vi "Alias.vi"() -> ()   [LabVIEW 2024]
uses:
  ASW/Source/DigitalThreadServices/DataStoreClient.LabVIEW/source/API/Metadata/Extension.ctl
  ASW/Source/DigitalThreadServices/DataStoreClient.LabVIEW/source/API/Metadata/NI Metadata Types.lvlib
  ASW/Source/DigitalThreadServices/DataStoreClient.LabVIEW/source/API/Metadata/Operator.ctl
  ASW/Source/DigitalThreadServices/DataStoreClient.LabVIEW/source/API/Metadata Store V1/NI Metadata Store V1 Client.lvlib
  ASW/Source/DigitalThreadServices/DataStoreClient.LabVIEW/source/API/Data Store V1/NI Data Store V1 Client.lvlib
  ASW/Source/DigitalThreadServices/DataStoreClient.LabVIEW/source/API/Metadata/Outcome.ctl
  ASW/Source/DigitalThreadServices/DataStoreClient.LabVIEW/source/API/Data Store V1/Test Result.ctl
  ASW/Source/DigitalThreadServices/DataStoreClient.LabVIEW/source/API/Metadata/Alias Target Type.ctl
  ASW/Source/DigitalThreadServices/DataStoreClient.LabVIEW/source/API/Metadata Store V1/Create Alias (Metadata - Operator).vi
  ASW/Source/DigitalThreadServices/DataStoreClient.LabVIEW/source/API/Metadata Store V1/Create Operator.vi
  ASW/Source/DigitalThreadServices/DataStoreClient.LabVIEW/source/API/Metadata Store V1/Get Operator.vi
  ASW/Source/DigitalThreadServices/DataStoreClient.LabVIEW/source/API/Metadata/Error Information.ctl
  ASW/Source/DigitalThreadServices/DataStoreClient.LabVIEW/source/API/Metadata/Alias.ctl
panel:
  in  "Operator Info":cluster{"Name":string, "Alias":string}[](array[cluster])=[{"Name"="Jane Doe", "Alias"="primary_operator"}, {"Name"="John Smith", "Alias"="secondary_operator"}]
  out "query aliases results":T1[](array[typedef])
  out "get alias results":T1
  out "log":string
  out "error out":errorcluster
  # "Using Aliases\n\nThis example shows how to use the datastore API to...\n- Create aliases for metadata\n- Use created aliases\n- Retrieve aliases\n- Delete aliases"
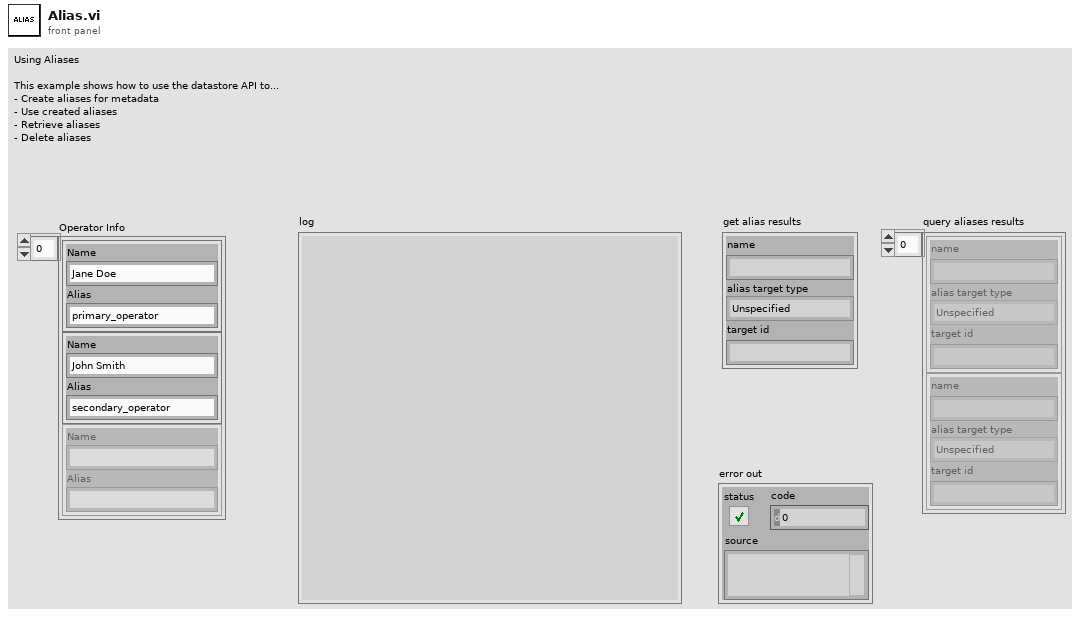
[diagram p1: front panel]
types:
  T1 = typedef "NI Metadata Types.lvlib/Alias.ctl" = cluster{"name":string, "alias target type":T2, "target id":string}
  T2 = typedef "NI Metadata Types.lvlib/Alias Target Type.ctl" = enum32{"Unspecified", "UUT Instance", "UUT", "Hardware Item", "Software Item", "Operator", "Test Description", "Test", "Test Station", "Test Adapter"}
  T3 = enum16{"Create Aliases", "Use the Alias", "Retrieve Aliases", "Delete Aliases"}
  T4 = cluster{"value":string, "value":string, "value":string, "value":string, "value":string}
  T5 = typedef "NI Metadata Types.lvlib/Operator.ctl" = cluster{"name":string, "role":string, "id":string, "link":string, "extension":T6[], "schema id":string}
  T6 = typedef "NI Metadata Types.lvlib/Extension.ctl" = cluster{"name":string, "value":string}
  T7 = typedef "NI Data Store V1 Client.lvlib/Test Result.ctl" = cluster{"name":string, "start date time":timestamp, "end date time":timestamp, "outcome":T8, "error information":T9, "id":string, "uut instance id":string, "operator id":string, "test station id":string, "test description id":string, "software item ids":string[], "hardware item ids":string[], "test adapter ids":string[], "link":string, "extension":T6[], "schema id":string}
  T8 = typedef "NI Metadata Types.lvlib/Outcome.ctl" = enum32{"Unspecified", "Passed", "Failed", "Indeterminate"}
  T9 = typedef "NI Metadata Types.lvlib/Error Information.ctl" = cluster{"error code":i32, "message":string, "source":string}
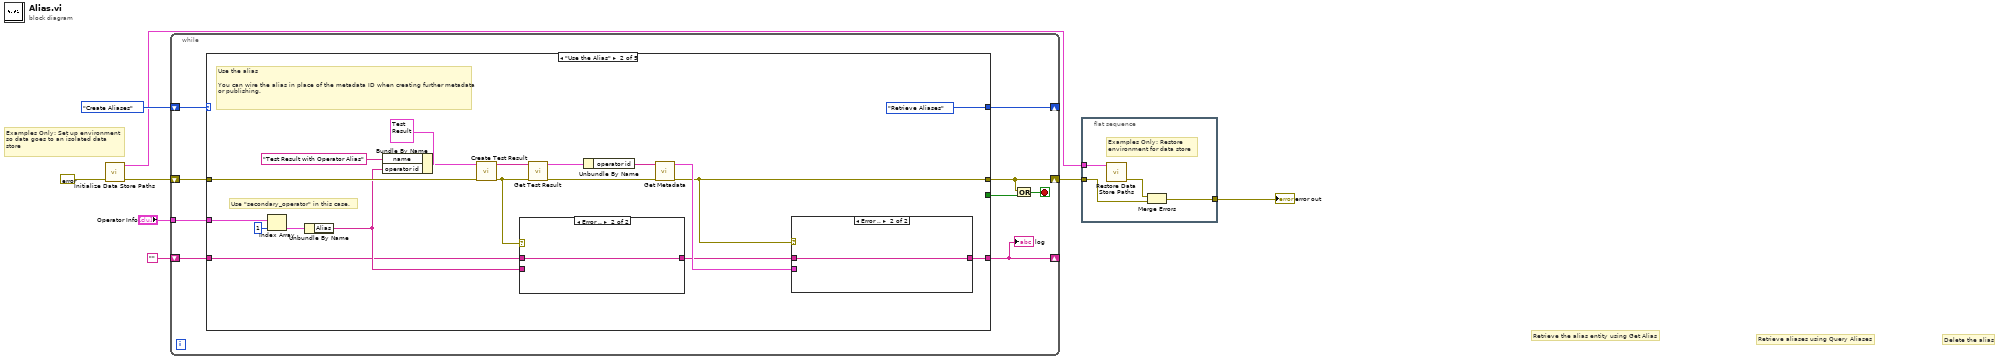
[diagram p0: block diagram]
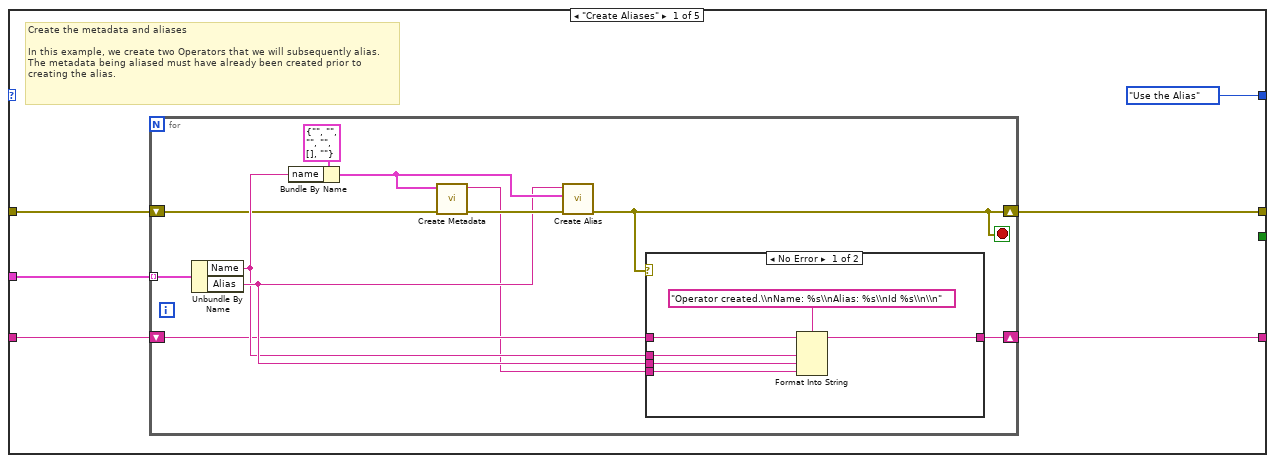
[diagram p2: hidden frame]
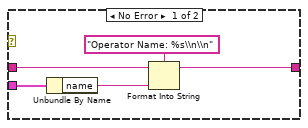
[diagram p4: hidden frame]
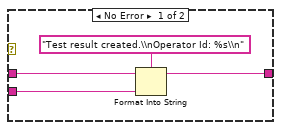
[diagram p5: hidden frame]
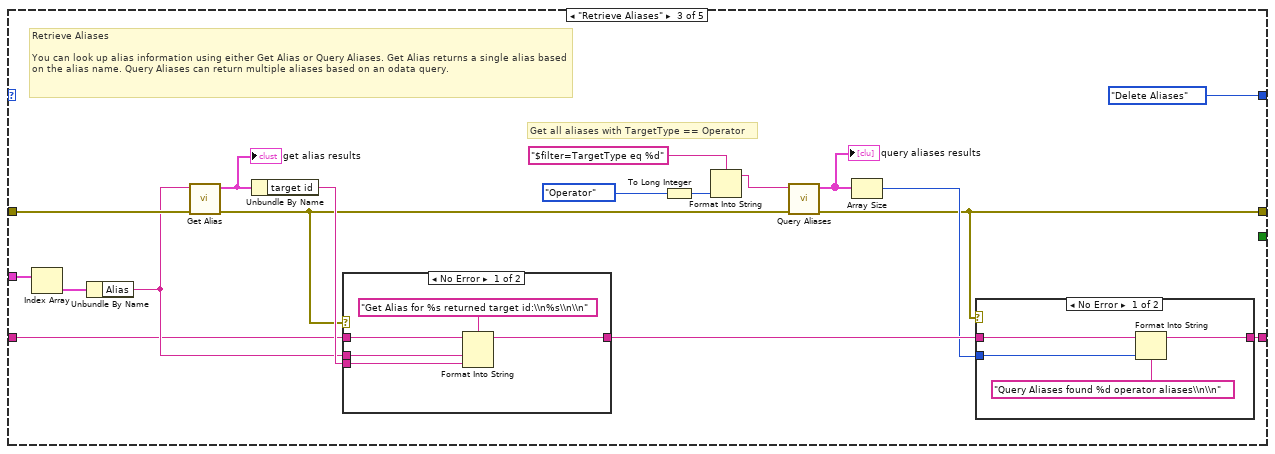
[diagram p6: hidden frame]
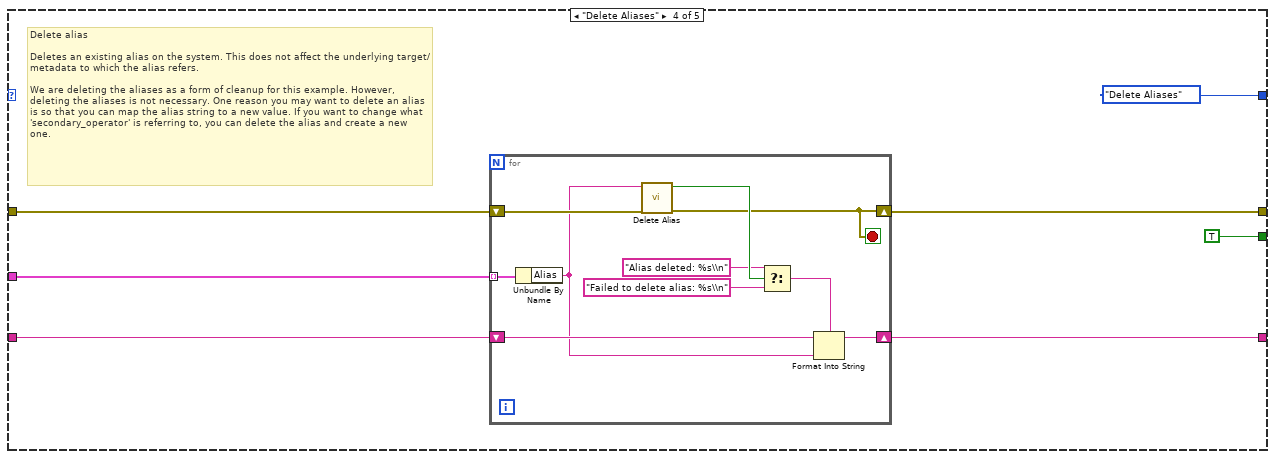
[diagram p9: hidden frame]
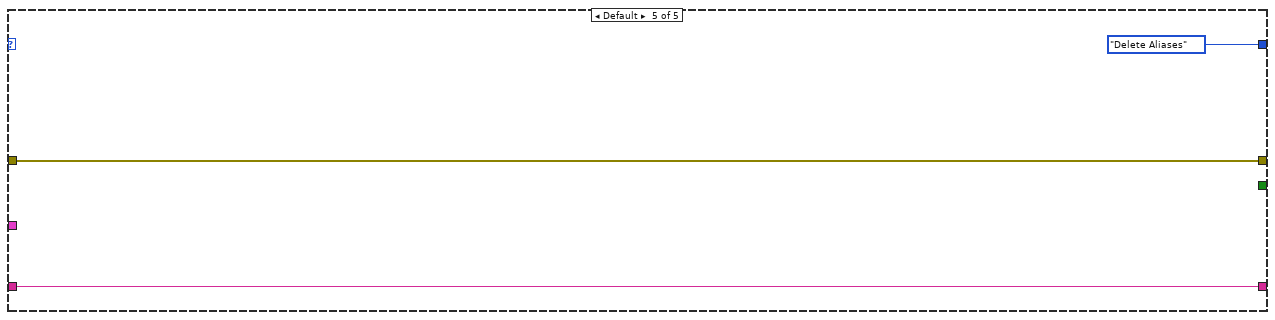
[diagram p10: hidden frame]
diagram:
  # "Examples Only: Set up environment\nso data goes to an isolated data\nstore"
  # "Delete the alias"
  # "Retrieve aliases using Query Aliases"
  # "Retrieve the alias entity using Get Alias"
  n1 = call "Initialize Data Store Paths.vi"("error in"=errorcluster {"status"=FALSE, "code"=0, "source"=""} ("error out")) -> ("error out"=w4:errorcluster, "original values"=w3:T4)  [unwired: 9 in]
  n2 = while {
    shift-right: [w12] -> _
    shift-left: T3."Create Aliases" -> [w17]
    shift-right: [w13] -> _
    shift-left: "" ("log") -> [w15]
    tunnel: "Operator Info" -> [w16]
    shift-right: [w11] -> w2
    shift-left: w4 -> [w14]
    stop <- w9 stop-if-true
    n3 = case shown="\"Use the Alias\"" w17 {
      tunnel: w16 -> [w23 w51 w79 w105 _]
      tunnel: [w22 w43 w73 w101 w120] -> w11
      tunnel: w15 -> [w21 w47 w76 w107 w119]
      tunnel: [w20 w45 w75 w104 w119] -> w13
      tunnel: w14 -> [w19 w52 w80 w106 w120]
      tunnel: [T3."Use the Alias" T3."Retrieve Aliases" T3."Delete Aliases" T3."Delete Aliases" T3."Delete Aliases"] -> w12
      tunnel: [_ _ _ TRUE _] -> w10
      frame "Create Aliases" {
        # "Create the metadata and aliases\n\nIn this example, we create two Operators that we will subsequently alias. The metadata being aliased must have already been created prior to creating the alias."
        n4 = for {
          shift-right: [w25] -> w22
          shift-left: w19 -> [w26]
          tunnel: w23 -> [w31] mode=indexing
          shift-right: [w27] -> w20
          shift-left: w21 -> [w28]
          stop <- w25 stop-if-true
          n5 = Unbundle By Name(w31) -> ("Name"=w29:string, "Alias"=w30:string)
          n6 = Bundle By Name(cluster=T5 {"name"="", "role"="", "id"="", "link"="", "extension"=[], "schema id"=""} ("operator metadata"), "name"=w29) -> (w33:T5)
          n7 = call-poly "Create Metadata.vi"("error in"=w26, "operator metadata"=w33) -> ("error out"=w34:errorcluster, "operator id"=w24:string)  [unwired: 8 in]
          n8 = call-poly "Create Alias.vi"("error in"=w34, "operator"=w33, "alias name"=w30) -> ("error out"=w25:errorcluster)  [unwired: 7 in, 1 out]
          n9 = case shown="No Error" w25 {
            tunnel: w30 -> [w40 _]
            tunnel: w29 -> [w39 _]
            tunnel: w28 -> [w38 w41]
            tunnel: [w37 w41] -> w27
            tunnel: w24 -> [w36 _]
            frame No Error {
              n10 = Format Into String(format string="Operator created.\\nName: %s\\nAlias: %s\\nId %s\\n\\n", initial string=w38, w39, w40, w36) -> (resulting string=w37:string)  [unwired: 1 in, 1 out]
            }
            frame Error {
            }
          }
        }
      }
      frame "Use the Alias" {
        # "Use the alias\n\nYou can wire the alias in place of the metadata ID when creating further metadata or publishing."
        # "Use \"secondary_operator\" in this case."
        n11 = Index Array(array=w51, index=1) -> (element=w49:cluster{"Name":string, "Alias":string})
        n12 = Unbundle By Name(w49) -> ("Alias"=w48:string)
        n13 = Bundle By Name(cluster=T7 {"name"="", "start date time"=timestamp(0 s since 1904-01-01), "end date time"=timestamp(0 s since 1904-01-01), "outcome"=enum."Unspecified", "error information"={"error code"=0, "message"="", "source"=""}, "id"="", "uut instance id"="", "operator id"="", "test station id"="", "test description id"="", "software item ids"=[], "hardware item ids"=[], "test adapter ids"=[], "link"="", "extension"=[], "schema id"=""} ("test result"), "name"="Test Result with Operator Alias" ("test result name"), "operator id"=w48) -> (w57:T7)
        n14 = call "Create Test Result.vi"("error in"=w52, "test result"=w57) -> ("error out"=w44:errorcluster, "test result id"=w60:string)  [unwired: 8 in]
        n15 = case shown="Error .." w44 {
          tunnel: w48 -> [w69 _]
          tunnel: w47 -> [w68 w71]
          tunnel: [w67 w71] -> w46
          frame No Error {
            n16 = Format Into String(format string="Test result created.\\nOperator Id: %s\\n", initial string=w68, w69) -> (resulting string=w67:string)  [unwired: 1 in, 1 out]
          }
          frame Error {
          }
        }
        n17 = call "Get Test Result.vi"("error in"=w44, "test result id"=w60) -> ("error out"=w56:errorcluster, "test result"=w55:T7)  [unwired: 8 in]
        n18 = Unbundle By Name(w55) -> ("operator id"=w54:string)
        n19 = call-poly "Get Metadata.vi"("error in"=w56, "operator id"=w54) -> ("error out"=w43:errorcluster, "operator metadata"=w53:T5)  [unwired: 8 in]
        n20 = case shown="Error .." w43 {
          tunnel: w53 -> [w63 _]
          tunnel: w46 -> [w62 w66]
          tunnel: [w61 w66] -> w45
          frame No Error {
            n21 = Unbundle By Name(w63) -> ("name"=w65:string)
            n22 = Format Into String(format string="Operator Name: %s\\n\\n", initial string=w62, w65) -> (resulting string=w61:string)  [unwired: 1 in, 1 out]
          }
          frame Error {
          }
        }
      }
      frame "Retrieve Aliases" {
        # "Get all aliases with TargetType == Operator"
        # "Retrieve Aliases\n\nYou can look up alias information using either Get Alias or Query Aliases. Get Alias returns a single alias based on the alias name. Query Aliases can return multiple aliases based on an odata query."
        n23 = Index Array(array=w79) -> (element=w78:cluster{"Name":string, "Alias":string})  [unwired: 1 in]
        n24 = Unbundle By Name(w78) -> ("Alias"=w77:string)
        n25 = call "Get Alias.vi"("error in"=w80, "alias name"=w77) -> ("error out"=w74:errorcluster, "alias"=w81:T1)  [unwired: 8 in]
        "get alias results" <- w81
        n26 = Unbundle By Name(w81) -> ("target id"=w82:string)
        n27 = case shown="No Error" w74 {
          tunnel: [w99 w100] -> w89
          tunnel: w82 -> [w98 _]
          tunnel: w77 -> [w97 _]
          tunnel: w76 -> [w96 w100]
          frame No Error {
            n28 = Format Into String(format string="Get Alias for %s returned target id:\\n%s\\n\\n" ("odata query"), initial string=w96, w97, w98) -> (resulting string=w99:string)  [unwired: 1 in, 1 out]
          }
          frame Error {
          }
        }
        n29 = To Long Integer(number=Alias_Target_Type."Operator" ("alias target type")) -> (32bit integer=w87:i32)
        n30 = Format Into String(format string="$filter=TargetType eq %d" ("odata query"), w87) -> (resulting string=w88:string)  [unwired: 2 in, 1 out]
        n31 = call "Query Aliases.vi"("error in"=w74, "odata query"=w88) -> ("error out"=w73:errorcluster, "aliases"=w83:T1[])  [unwired: 8 in]
        "query aliases results" <- w83
        n32 = Array Size(array=w83) -> (size(s)=w84:i32)
        n33 = case shown="No Error" w73 {
          tunnel: w89 -> [w93 w94]
          tunnel: w84 -> [w92 _]
          tunnel: [w91 w94] -> w75
          frame No Error {
            n34 = Format Into String(format string="Query Aliases found %d operator aliases\\n\\n" ("odata query"), initial string=w93, w92) -> (resulting string=w91:string)  [unwired: 1 in, 1 out]
          }
          frame Error {
          }
        }
      }
      frame "Delete Aliases" {
        # "Delete alias\n\nDeletes an existing alias on the system. This does not affect the underlying target/metadata to which the alias refers.\n\nWe are deleting the aliases as a form of cleanup for this example. However, deleting the aliases is not necessary. One reason you may want to delete an alias is so that you can map the alias string to a new value. If you want to change what 'secondary_operator' is referring to, you can delete the alias and create a new one."
        n35 = for {
          shift-right: [w108] -> w101
          shift-left: w106 -> [w116]
          tunnel: w105 -> [w115] mode=indexing
          shift-right: [w112] -> w104
          shift-left: w107 -> [w117]
          stop <- w108 stop-if-true
          n36 = Unbundle By Name(w115) -> ("Alias"=w114:string)
          n37 = call "Delete Alias.vi"("error in"=w116, "alias name"=w114) -> ("error out"=w108:errorcluster, "deleted"=w113:bool)  [unwired: 8 in]
          n38 = Select(t="Alias deleted: %s\\n" ("format string"), s=w113, f="Failed to delete alias: %s\\n" ("format string")) -> (s? t:f=w109:string)
          n39 = Format Into String(format string=w109, initial string=w117, w114) -> (resulting string=w112:string)  [unwired: 1 in, 1 out]
        }
      }
      frame Default {
      }
    }
    "log" <- w13
    n40 = Or(x=w11, y=w10) -> (x .or. y?=w9:bool)
  }
  n41 = flat-sequence {
    tunnel: w3 -> [w124]
    tunnel: w2 -> [w122]
    tunnel: [w121] -> w1
    frame #0 {
      # "Examples Only: Restore\nenvironment for data store"
      n42 = call "Restore Data Store Paths.vi"("original values"=w124) -> ("error out"=w123:errorcluster)  [unwired: 10 in]
      n43 = Merge Errors(w123, w122) -> (w121:errorcluster)
    }
  }
  "error out" <- w1
